vi "Get Class Path.vi"(11 "Base Class Name":string) -> (2 "Success?":bool, 3 "Path":path)   [LabVIEW 2019, in "ClassLoader.lvlib"]
doc: "Return path for the given class.\n\nThis VI does not automatically load data. Front-load before calling this VI!"
uses:
  ClassLoader.lvlib
  Sub/Cache/Cache_Path Global.vi
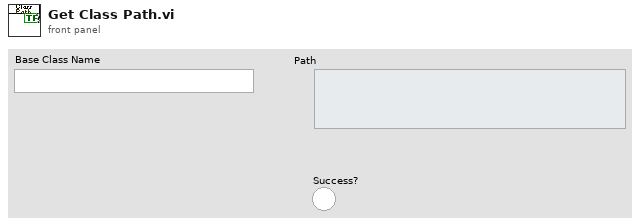
[diagram p1: front panel]
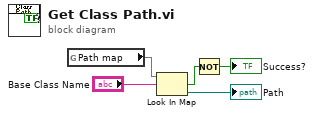
[diagram p0: block diagram]
diagram:
  n1 = global read "Cache_Path Global.vi" "Path map"() -> (w3:map{string, path})
  n2 = Look In Map(map=w3, key="Base Class Name") -> (key not found?=w2:bool, value=→"Path":path)  [unwired: 1 in]
  n3 = Not(x=w2) -> (.not. x?=→"Success?":bool)
